vi "UsingArrays.vi"() -> ()   [LabVIEW 2018]
panel:
  in  "index":i32
  out "element":dbl
  out "size(s)":i32
  in  "Array":dbl[](array[numeric])
  out "Array 2":dbl[](array[slide]) scale=0.0..10.0
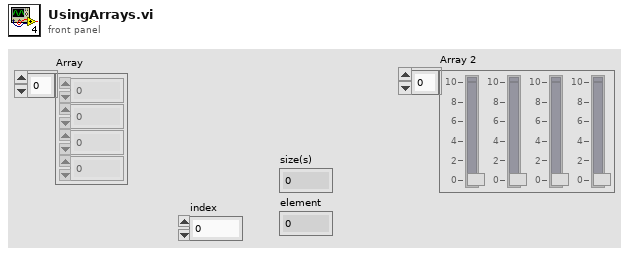
[diagram p1: front panel]
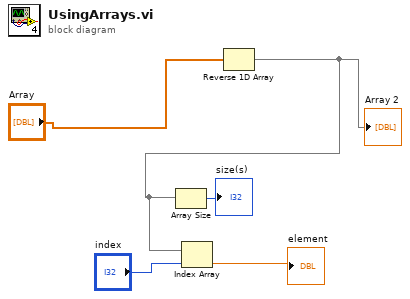
[diagram p0: block diagram]
diagram:
  n1 = Reverse 1D Array(array="Array") -> (reversed array=w1:dbl[])
  "Array 2" <- w1
  n2 = Array Size(array=w1) -> (size(s)=→"size(s)":i32)
  n3 = Index Array(array=w1, index="index") -> (element=→"element":dbl)
